vi "PropertyListToScript.vi"(9 "NewVal":string[](array[string]), 10 "VI Properties":refnum<vi>, 11 "TreeControl in":refnum<vi>) -> (3 "Script":string)   [LabVIEW 2019, in "VIPropertyPicker.lvlib"]
uses:
  VIPropertyPicker.lvlib
  c00798a1-a550-43e0-9540-3b7af162c467.vi
  lib/UI/TreeControl/TreeControlLib.lvlib
  lib/SetGetControlValue/SetGetControlValue.lvlib
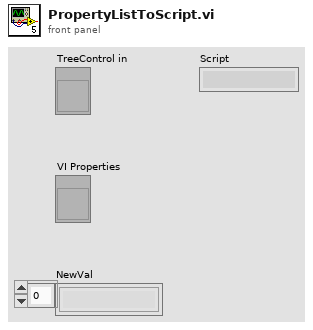
[diagram p1: front panel]
types:
  T1 = cluster{"Closed Nodes":string[], "Selection":string[], "Defer Panel Update":bool, "FocusItem":string}
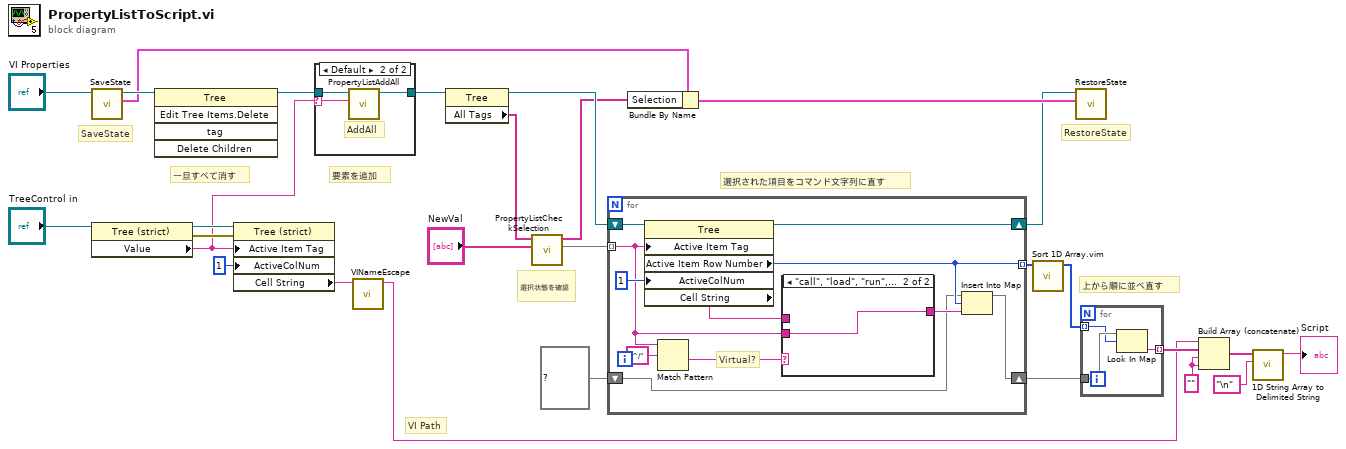
[diagram p0: block diagram]
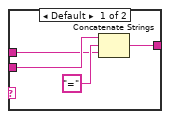
[diagram p3: hidden frame]
diagram:
  w3 = "" ("element")
  # "選択状態を確認"
  # "選択された項目をコマンド文字列に直す"
  # "上から順に並べ直す"
  # "VI Path"
  # "要素を追加"
  # "RestoreState"
  # "SaveState"
  # "一旦すべて消す"
  n1 = call "SaveState.vi"("TreeControl in"="VI Properties") -> ("State"=w17:T1, "TreeControl out"=w18:refnum<vi>)  [unwired: 8 in, 1 out]
  n2 = property class="Tree (strict)"(reference="TreeControl in") -> (reference out=w12:refnum<vi>, error out=w11:errorcluster, "Value"=w10:string)  [unwired: 1 in]
  n3 = invoke class="Tree" method="Edit Tree Items.Delete"(reference=w18) -> (reference out=w27:refnum<vi>)  [unwired: 4 in, 4 out]
  n4 = property class="Tree (strict)"(reference=w12, error in=w11, "Active Item Tag"=w10, "ActiveColNum"=1 ("Active Cell:Active Column Number")) -> ("Cell String"=w4:string)  [unwired: 2 out]
  n5 = case shown="Default" w10 {
    selector: w10 -> [_ w31]
    tunnel: w27 -> [w29 w30]
    tunnel: [w29 w32] -> w26
    frame "" {
    }
    frame Default {
      # "AddAll"
      n6 = call "PropertyListAddAll.vi"("VITag"=w31, "PropertyList in"=w30) -> ("PropertyList out"=w32:refnum<vi>)  [unwired: 9 in]
    }
  }
  n7 = call "VINameEscape.vi"("label"=w4) -> ("escaped string"=w1:string)  [unwired: 10 in]
  n8 = property class="Tree"(reference=w26) -> (reference out=w25:refnum<vi>, "All Tags"=w15:string[])  [unwired: 1 in, 1 out]
  n9 = call "PropertyListCheckSelection.vi"("Selectrion in"="NewVal", "All Tags"=w15) -> ("Children removed"=w14:set{string}, "Selection out"=w13:string[])  [unwired: 8 in]
  n10 = for {
    tunnel: w14 -> [w38] mode=indexing
    shift-right: [w36] -> w23
    shift-left: map{i32, string} {} ("map") -> [w33]
    tunnel: [w35] -> w6 mode=indexing
    shift-right: [w34] -> w19
    shift-left: w25 -> [w43]
    # "Virtual?"
    n11 = property class="Tree"(reference=w43, "Active Item Tag"=w38, "ActiveColNum"=1 ("Active Cell:Active Column Number")) -> (reference out=w34:refnum<vi>, "Active Item Row Number"=w35:i32, "Cell String"=w39:string)  [unwired: 1 in, 1 out]
    n12 = Match Pattern(string=w38, regular expression="^/") -> (after substring=w41:string)  [unwired: 1 in, 3 out]
    n13 = case shown="\"call\", \"load\", \"run\", \"stop\"" w41 {
      tunnel: [w44 w48] -> w37
      tunnel: w38 -> [w47 w48]
      tunnel: w39 -> [w45 _]
      frame Default {
        n14 = Concatenate Strings(w47, "=" ("string"), w45) -> (w44:string)
      }
      frame "call", "load", "run", "stop" {
      }
    }
    n15 = Insert Into Map(map in=w33, key=w35, value=w37) -> (map out=w36:map{i32, string})  [unwired: 2 out]
  }
  n16 = Bundle By Name(cluster=w17, "Selection"=w13) -> (w20:T1)
  n17 = call "Sort 1D Array.vim"("unsorted array"=w6) -> ("sorted array"=w24:i32[])  [unwired: 10 in]
  n18 = call "RestoreState.vi"("State"=w20, "TreeControl in"=w19) -> ()  [unwired: 8 in, 2 out]
  n19 = for {
    tunnel: w24 -> [w50] mode=indexing
    tunnel: w23 -> [w51]
    tunnel: [w49] -> w22 mode=indexing
    n20 = Look In Map(map=w51, key=w50) -> (value=w49:string)  [unwired: 1 in, 1 out]
  }
  n21 = Build Array (concatenate)(w1, w22, w3, w3) -> (w5:string[])
  n22 = call <vilib>:"1D String Array to Delimited String.vi"("delimiter"="\n", "string array"=w5) -> ("delimited string"=→"Script":string)  [unwired: 9 in]
